vi "Comm D2XX.vi"(5 "Motion Code":string="\u0004", 6 "error in (no error)":errorcluster, 8 "steps/sec":u32=20, 9 "motor rotation":bool caption="motor direction", 10 "Steps":dbl=1.0, 11 "Motor":T1) -> (1 "Estimated time [sec]":dbl, 2 "Read Buffer Out":string, 3 "device found":bool, 4 "error out":errorcluster)   [LabVIEW 2014, in "AISAS motor.lvclass"]
uses:
  AISAS motor.lvclass
  Controls/motor.ctl
panel:
  out "Read B in INT":u8
  in  "error in (no error) 2":errorcluster
  out "motor":string
  out "motor rotation 2":bool caption="motor direction"
  in  "bytes  to read":i32=1
  out "sec":ext
  out "Bytes Read":u32
  out "velocity":string
  out "rotation":string
  out "steps High B":string
  out "steps Low B":string="d"
  out "Device Description":string
  in  "Device Index":u32
  # "Time [sec]"
  # "roration motor - left - v smere  hod. ruciciek\n                       opt. rychlost 50steps/s"
  # "difuser - right - open difuser\n      6000 steps total\nCLOSE - LEFT\noptimal speed - 60steps/s\nMK+JR, 20140305 prevod 1:4.375"
  # "velocity = 730,88/steps.p.sec"
  # "left"
  # "Slow = 0"
  # "Fast = 365"
  # "OFFF objective lens klesaju hodnotyy"
  # "right"
  # "ON  ide smerom hore rychlost 60 zdravy stred"
  # "Rotation motor: smer left otaca filter modul doprava v pohlade smerom odspodu\nrychlost 10steps/s"
  # "Zmena od 28-MAR-2013, Jaro doplnil inteligentne snimace a vynovil elektroniku motorov.\nTeraz je poradie prikazu: vyber motora ->kod pohybu -> Dolny byte -> horny byte -> smer -> rychlost\nmotory dostali novy kod: DIFF=01, OBJ.LENS=02,ROT=03"
  # "Uprava 25-AUG-2013: OBJ. LENS=02\nDIFF = 01\nROTATION = 00\n!!!!"
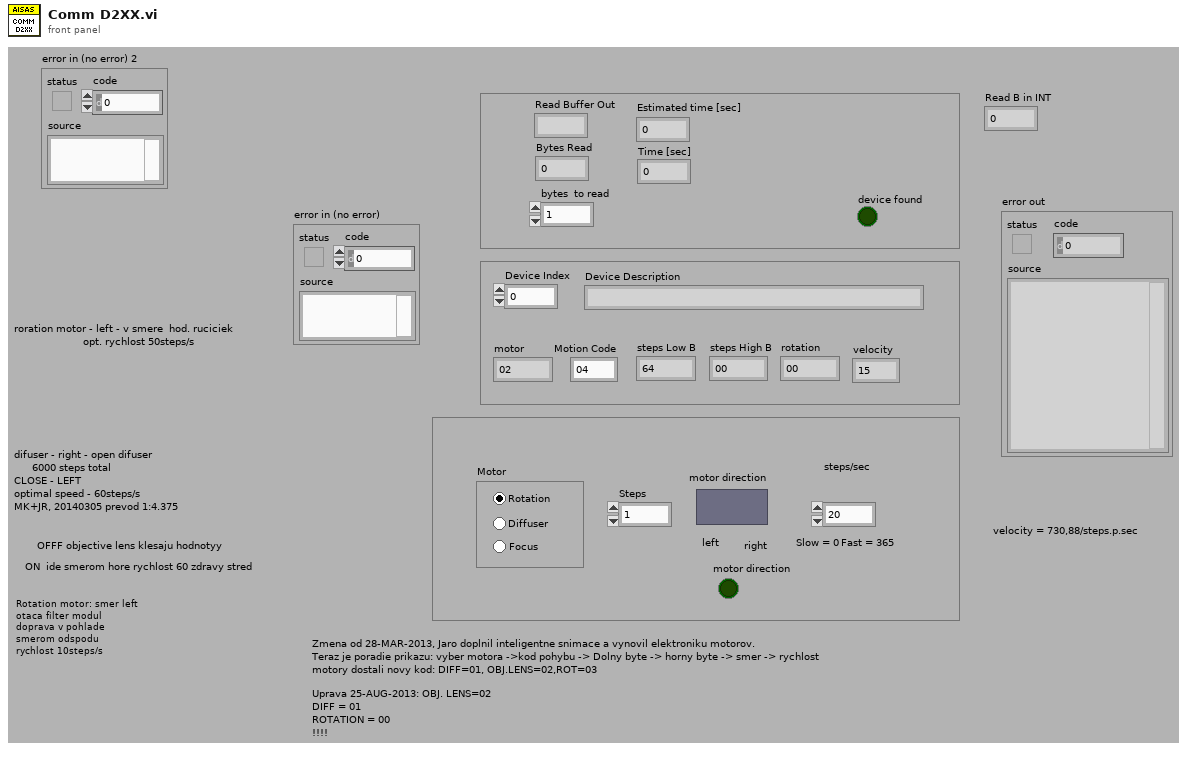
[diagram p1: front panel]
types:
  T1 = typedef "motor.ctl" = enum32{"Rotation", "Diffuser ", "Focus"}
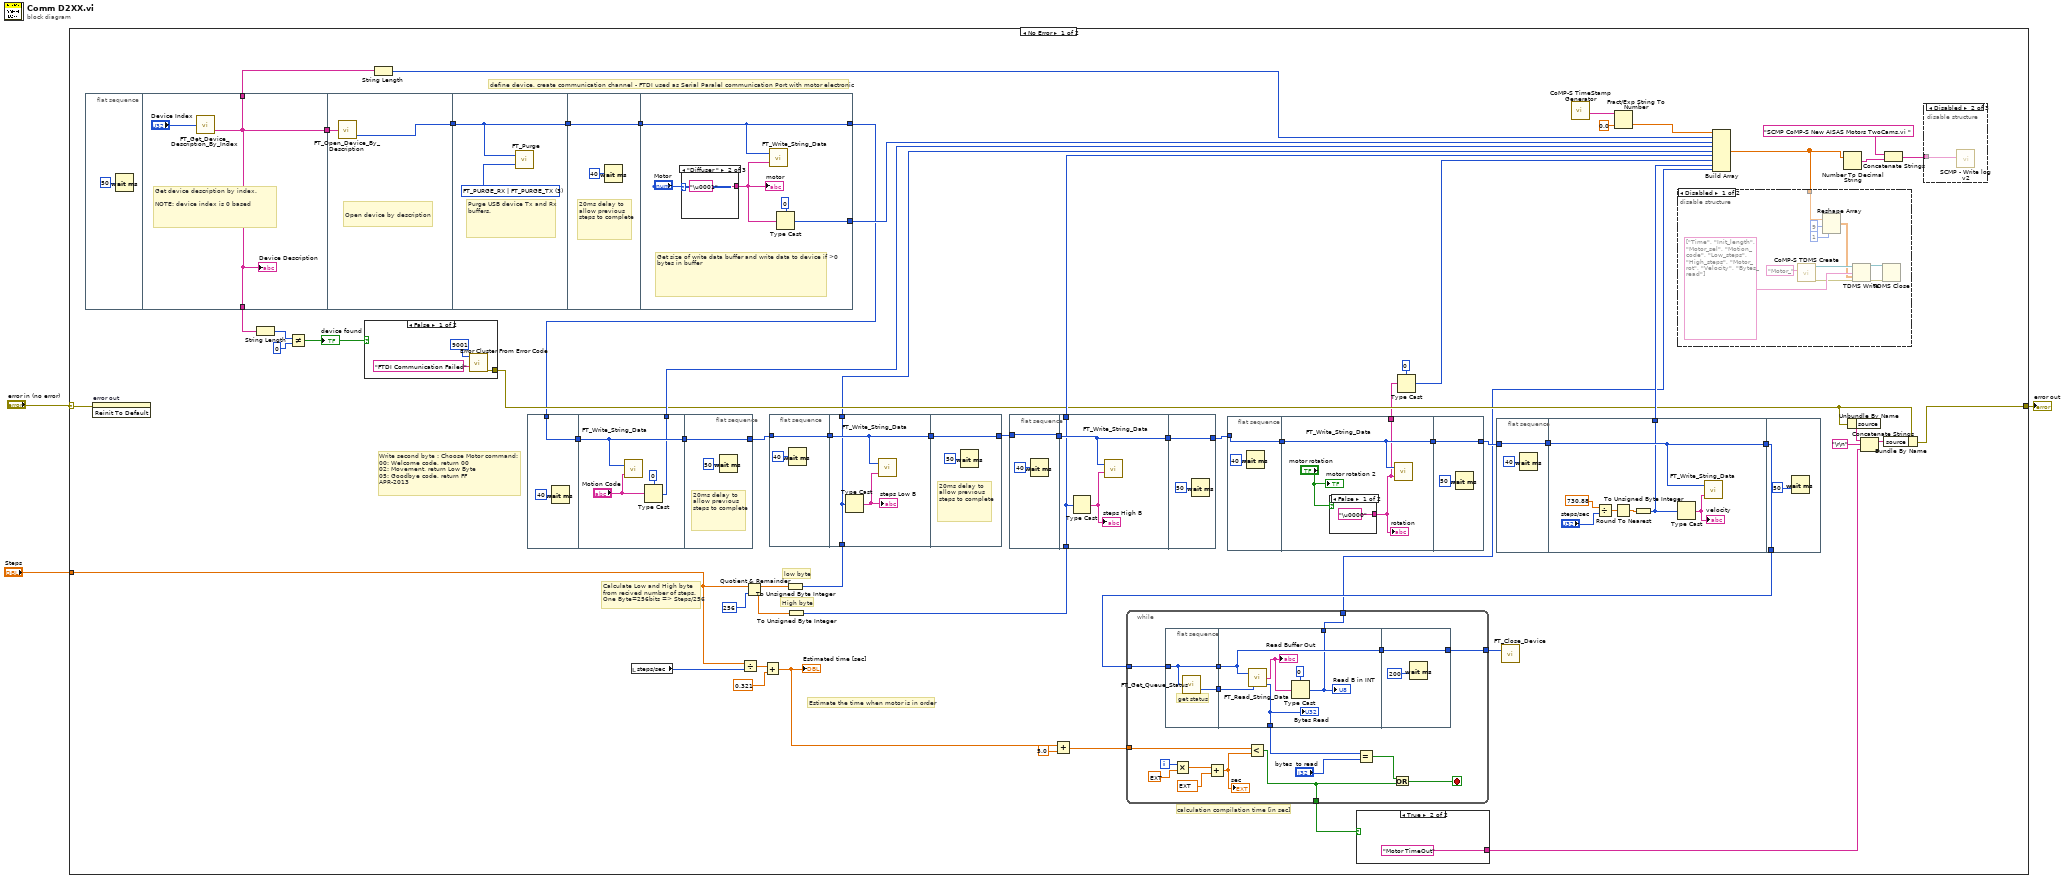
[diagram p0: block diagram]
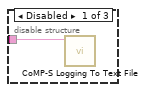
[diagram p3: hidden frame]
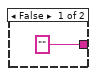
[diagram p5: hidden frame]
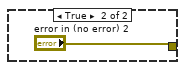
[diagram p6: hidden frame]
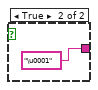
[diagram p7: hidden frame]
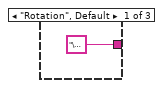
[diagram p8: hidden frame]
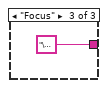
[diagram p9: hidden frame]
diagram:
  n1 = case shown="No Error" "error in (no error)" {
    selector: "error in (no error)" -> [w6 w171]
    tunnel: [w4 w171] -> w3
    tunnel: "Steps" -> [w28 _]
    frame No Error {
      # "Estimate the time when motor is in order"
      # "Calculate Low and High byte\nfrom recived number of steps. \nOne Byte=256bits => Steps/256"
      # "Write second byte : Choose Motor command:\n00: Welcome code, return 00\n02: Movement, return Low Byte\n05: Goodbye code, return FF\nAPR-2013"
      # "define device, create communication channel - FTDI used as Serial Paralel communication Port with motor electronic"
      # "High byte"
      # "low byte"
      # "calculation compilation time [in sec]"
      n2 = flat-sequence {
        tunnel: [w155] -> w66
        tunnel: [w155] -> w39
        tunnel: [w155] -> w26
        tunnel: [w158] -> w65
        tunnel: w66 -> [w157]
        tunnel: [w159] -> w64
        tunnel: w65 -> [w159]
        tunnel: [w161] -> w63
        tunnel: w64 -> [w161]
        tunnel: [w167] -> w7
        tunnel: w63 -> [w167]
        tunnel: [w164] -> w24
        frame #0 {
          n3 = Wait (ms)(milliseconds to wait=u32 50) -> ()  [unwired: 1 out]
        }
        frame #1 {
          # "Get device description by index.\n\nNOTE: device index is 0 based"
          n4 = call "FT_Get_Device_Description_By_Index.vi"("Device Index"="Device Index") -> ("Device Description"=w155:string)  [unwired: 1 out]
          "Device Description" <- w155
        }
        frame #2 {
          # "Open device by description"
          n5 = call "FT_Open_Device_By_Description.vi"("Device Description"=w157) -> ("Handle"=w158:u32)  [unwired: 1 out]
        }
        frame #3 {
          w160 = u32 3 items=["FT_PURGE_RX"=1, "FT_PURGE_TX"=2, "FT_PURGE_RX | FT_PURGE_TX"=3] ("Purge Flags")
          # "Purge USB device Tx and Rx buffers."
          n6 = call "FT_Purge.vi"("Purge Flags"=w160, "Handle"=w159) -> ()  [unwired: 1 out]
        }
        frame #4 {
          # "20ms delay to allow previous steps to complete"
          n7 = Wait (ms)(milliseconds to wait=u32 40) -> ()  [unwired: 1 out]
        }
        frame #5 {
          # "Get size of write data buffer and write data to device if >0 bytes in buffer"
          n8 = case shown="\"Diffuser \"" "Motor" {
            tunnel: ["\u0000" "\u0001" "\u0002"] -> w166
            frame "Rotation", Default {
            }
            frame "Diffuser " {
            }
            frame "Focus" {
            }
          }
          "motor" <- w166
          n9 = call "FT_Write_String_Data.vi"("Buffer"=w166, "Handle"=w167) -> ()  [unwired: 2 out]
          n10 = Type Cast(type=u8 0 ("default (0 U32)"), x=w166) -> (*(type *) &x=w164:u8)
        }
      }
      n11 = invoke on="error out" class="Clust (strict)" method="Reinit To Default"(error in=w6) -> ()  [unwired: 2 in, 3 out]
      n12 = String Length(string=w39) -> (length=w38:i32)
      n13 = Not Equal?(x=w38, y=0) -> (x != y?=w36:bool)
      "device found" <- w36
      n14 = case shown="False" w36 {
        tunnel: [w81 "error in (no error) 2"] -> w17
        frame False {
          n15 = call <vilib>:"Error Cluster From Error Code.vi"("error message (\"\")"="FTDI Communication Failed" ("error message (\"\")"), "error code (0)"=9001) -> ("error out"=w81:errorcluster)  [unwired: 7 in]
        }
        frame True {
        }
      }
      n16 = String Length(string=w26) -> (length=w25:i32)
      n17 = flat-sequence {
        tunnel: [w147] -> w62
        tunnel: w7 -> [w147]
        tunnel: w62 -> [w151]
        tunnel: [w151] -> w61
        tunnel: [w148] -> w23
        tunnel: [w152] -> w52
        tunnel: w61 -> [w152]
        frame #0 {
          n18 = Wait (ms)(milliseconds to wait=u32 40) -> ()  [unwired: 1 out]
        }
        frame #1 {
          n19 = call "FT_Write_String_Data.vi"("Buffer"="Motion Code", "Handle"=w151) -> ()  [unwired: 2 out]
          n20 = Type Cast(type=u8 0 ("default (0 U32)"), x="Motion Code") -> (*(type *) &x=w148:u8)
        }
        frame #2 {
          # "20ms delay to allow previous steps to complete"
          n21 = Wait (ms)(milliseconds to wait=u32 50) -> ()  [unwired: 1 out]
        }
      }
      n22 = local read "steps/sec"() -> (w27:u32)
      n23 = Divide(x=w28, y=w27) -> (x/y=w41:dbl)
      n24 = Quotient & Remainder(x=w28, y=256) -> (x-y*floor(x/y)=w43:dbl, floor(x/y)=w45:dbl)
      n25 = Add(x=w41, y=0.321) -> (x+y=w34:dbl)
      "Estimated time [sec]" <- w34
      n26 = flat-sequence {
        tunnel: [w139] -> w60
        tunnel: w52 -> [w139]
        tunnel: [w143] -> w59
        tunnel: w42 -> [w141]
        tunnel: w60 -> [w143]
        tunnel: [w141] -> w8
        tunnel: [w144] -> w51
        tunnel: w59 -> [w144]
        frame #0 {
          n27 = Wait (ms)(milliseconds to wait=u32 40) -> ()  [unwired: 1 out]
        }
        frame #1 {
          n28 = Type Cast(x=w141) -> (*(type *) &x=w142:string)  [unwired: 1 in]
          "steps Low B" <- w142
          n29 = call "FT_Write_String_Data.vi"("Buffer"=w142, "Handle"=w143) -> ()  [unwired: 2 out]
        }
        frame #2 {
          # "20ms delay to allow previous steps to complete"
          n30 = Wait (ms)(milliseconds to wait=u32 50) -> ()  [unwired: 1 out]
        }
      }
      n31 = To Unsigned Byte Integer(number=w43) -> (unsigned 8bit integer=w42:u8)
      n32 = To Unsigned Byte Integer(number=w45) -> (unsigned 8bit integer=w44:u8)
      n33 = flat-sequence {
        tunnel: [w132] -> w58
        tunnel: w51 -> [w132]
        tunnel: [w136] -> w57
        tunnel: w44 -> [w134]
        tunnel: w58 -> [w136]
        tunnel: [w134] -> w22
        tunnel: [w137] -> w50
        tunnel: w57 -> [w137]
        frame #0 {
          n34 = Wait (ms)(milliseconds to wait=u32 40) -> ()  [unwired: 1 out]
        }
        frame #1 {
          n35 = Type Cast(x=w134) -> (*(type *) &x=w135:string)  [unwired: 1 in]
          "steps High B" <- w135
          n36 = call "FT_Write_String_Data.vi"("Buffer"=w135, "Handle"=w136) -> ()  [unwired: 2 out]
        }
        frame #2 {
          n37 = Wait (ms)(milliseconds to wait=u32 50) -> ()  [unwired: 1 out]
        }
      }
      n38 = Add(x=w34, y=5.0) -> (x+y=w33:dbl)
      n39 = while {
        tunnel: w48 -> [w101]
        tunnel: [w95] -> w47
        tunnel: w33 -> [w94]
        tunnel: [w86] -> w32
        tunnel: [w85] -> w13
        i -> [w89]
        stop <- w87 stop-if-true
        n40 = flat-sequence {
          tunnel: w101 -> [w102]
          tunnel: [w103] -> w100
          tunnel: [w102] -> w99
          tunnel: w100 -> [w109]
          tunnel: w99 -> [w107]
          tunnel: [w108] -> w97
          tunnel: [w107] -> w96
          tunnel: [w104] -> w85
          tunnel: w96 -> [w110]
          tunnel: [w110] -> w95
          frame #0 {
            # "get status"
            n41 = call "FT_Get_Queue_Status.vi"("Handle"=w102) -> ("Bytes Waiting"=w103:u32)  [unwired: 1 out]
          }
          frame #1 {
            n42 = call "FT_Read_String_Data.vi"("Handle"=w107, "Bytes To Read"=w109) -> ("Read Data"=w105:string, "Bytes Read"=w108:u32)  [unwired: 1 out]
            "Read Buffer Out" <- w105
            "Bytes Read" <- w108
            n43 = Type Cast(type=u8 0 ("default (0 U32)"), x=w105) -> (*(type *) &x=w104:u8)
            "Read B in INT" <- w104
          }
          frame #2 {
            n44 = Wait (ms)(milliseconds to wait=u32 200) -> ()  [unwired: 1 out]
          }
        }
        n45 = Multiply(x=w89, y=ext 0.2) -> (x*y=w92:ext)
        n46 = Add(x=w92, y=ext 0.32099999999999999999) -> (x+y=w88:ext)
        "sec" <- w88
        n47 = Less?(x=w94, y=w88) -> (x < y?=w86:bool)
        n48 = Equal?(x=w97, y="bytes  to read") -> (x = y?=w93:bool)
        n49 = Or(x=w93, y=w86) -> (x .or. y?=w87:bool)
      }
      n50 = flat-sequence {
        tunnel: [w124] -> w56
        tunnel: w50 -> [w124]
        tunnel: w56 -> [w127]
        tunnel: [w127] -> w55
        tunnel: [w125] -> w15
        tunnel: [w130] -> w49
        tunnel: w55 -> [w130]
        frame #0 {
          n51 = Wait (ms)(milliseconds to wait=u32 40) -> ()  [unwired: 1 out]
        }
        frame #1 {
          n52 = case shown="False" "motor rotation" {
            tunnel: ["\u0000" "\u0001"] -> w125
            frame False {
            }
            frame True {
            }
          }
          "rotation" <- w125
          n53 = call "FT_Write_String_Data.vi"("Buffer"=w125, "Handle"=w127) -> ()  [unwired: 2 out]
          "motor rotation 2" <- "motor rotation"
        }
        frame #2 {
          n54 = Wait (ms)(milliseconds to wait=u32 50) -> ()  [unwired: 1 out]
        }
      }
      n55 = case shown="True" w32 {
        tunnel: ["" "Motor TimeOut" ("error message (\"\")")] -> w9
        frame False {
        }
        frame True {
        }
      }
      n56 = Type Cast(type=u8 0 ("default (0 U32)"), x=w15) -> (*(type *) &x=w14:u8)
      n57 = flat-sequence {
        tunnel: [w112] -> w54
        tunnel: w49 -> [w112]
        tunnel: [w120] -> w53
        tunnel: w54 -> [w120]
        tunnel: [w114] -> w21
        tunnel: w53 -> [w121]
        tunnel: [w121] -> w48
        frame #0 {
          n58 = Wait (ms)(milliseconds to wait=u32 40) -> ()  [unwired: 1 out]
        }
        frame #1 {
          n59 = Divide(x=730.88, y="steps/sec") -> (x/y=w118:dbl)
          n60 = Round To Nearest(number=w118) -> (nearest integer value=w117:dbl)
          n61 = To Unsigned Byte Integer(number=w117) -> (unsigned 8bit integer=w114:u8)
          n62 = Type Cast(x=w114) -> (*(type *) &x=w119:string)  [unwired: 1 in]
          "velocity" <- w119
          n63 = call "FT_Write_String_Data.vi"("Buffer"=w119, "Handle"=w120) -> ()  [unwired: 2 out]
        }
        frame #2 {
          n64 = Wait (ms)(milliseconds to wait=u32 50) -> ()  [unwired: 1 out]
        }
      }
      n65 = call "FT_Close_Device.vi"("Handle"=w47) -> ()  [unwired: 1 out]
      n66 = call "CoMP-S TimeStamp Generator.vi"() -> ("date/time string"=w20:string)  [unwired: 10 in, 1 out]
      n67 = Fract/Exp String To Number(string=w20, default (0 dbl)=0.0 ("default (0 I32)")) -> (number=w18:dbl)  [unwired: 2 in, 1 out]
      n68 = Build Array(w18, w25, w24, w23, w8, w22, w14, w21, w13) -> (w12:dbl[])
      n69 = disable-structure shown="Disabled" {
        disable-tunnel: w12 -> [w67 _]
        frame Disabled {
          n70 = call "CoMP-S TDMS Create.vi"("Prefix"="Motor_") -> ("error out"=w74:errorcluster, "tdms file out"=w76:refnum<k34>)  [unwired: 7 in, 2 out]
          n71 = Reshape Array(w67, 9 ("dimension size"), 1 ("dimension size")) -> (w69:dbl[][])
          n72 = TDMS Write(0:w76, 7:string[] ["Time", "Init_length", "Motor_sel", "Motion_code", "Low_steps", "High_steps", "Motor_rot", "Velocity", "Bytes_read"] ("initialized array"), 9:w69, 11:w74) -> (4:w72:refnum<k34>, 15:w73:errorcluster)  [unwired: 2 in, 2 out]
          n73 = TDMS Close(8:w73, 11:w72) -> ()  [unwired: 2 out]
        }
        frame Enabled {
        }
      }
      n74 = Number To Decimal String(number=w12) -> (decimal integer string=w11:string[])  [unwired: 1 in]
      n75 = Unbundle By Name(w17) -> ("source"=w30:string)
      n76 = Concatenate Strings(w30, "\r\n", w9) -> (w31:string)
      n77 = Bundle By Name(cluster=w17, "source"=w31) -> (w4:errorcluster)
      n78 = Concatenate Strings("SCMP CoMP-S New AISAS Motors TwoCams.vi " ("string"), w11) -> (w5:string)
      n79 = disable-structure shown="Disabled" {
        disable-tunnel: w5 -> [w77 w78 _]
        frame Disabled {
          n80 = call "CoMP-S Logging To Text File.vi"("Input text"=w77) -> ()  [unwired: 10 in, 1 out]
        }
        frame Disabled {
          n81 = call "SCMP - Write log v2.vi"("data"=w78) -> ()  [unwired: 8 in, 3 out]
        }
        frame Enabled {
        }
      }
    }
    frame Error {
    }
  }
  "error out" <- w3
